vi "await_service_close.vi"(8 "error in (no error)":errorcluster, 11 "system.logging in":refnum<class "system.logging.lvclass">) -> (0 "error out":errorcluster, 3 "system.logging out":refnum<class "system.logging.lvclass">)   [LabVIEW 2021, in "system.logging.lvclass"]
uses:
  system.logging.lvclass
  system.logging.lvclass/system.logging.ctl
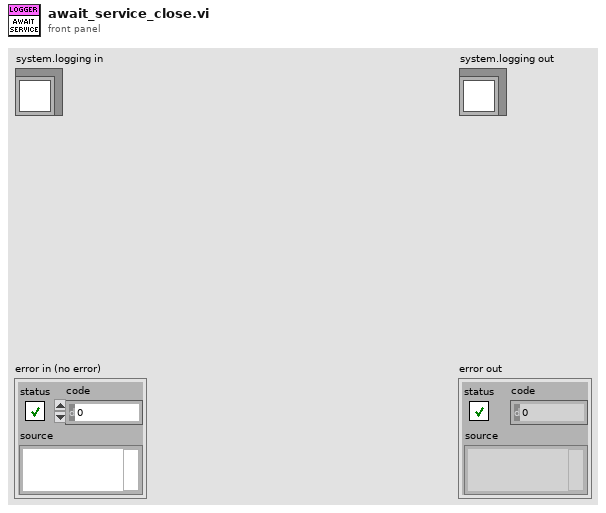
[diagram p1: front panel]
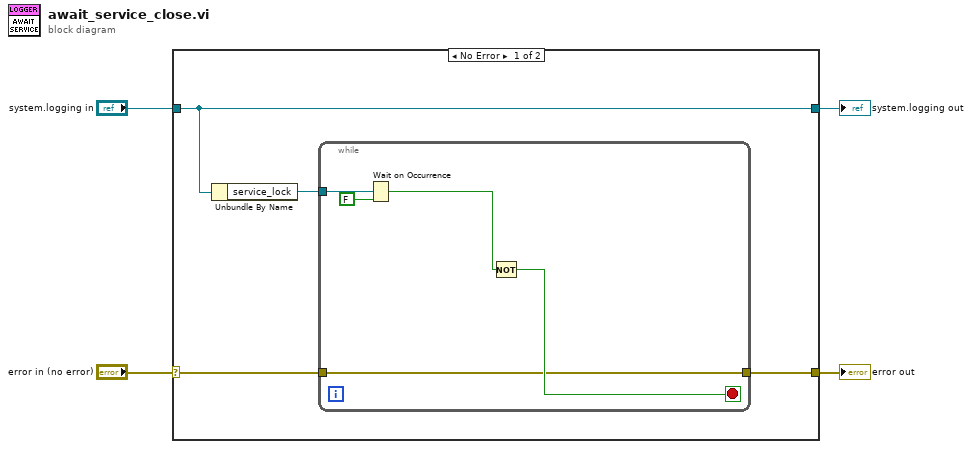
[diagram p0: block diagram]
diagram:
  n1 = case shown="No Error" "error in (no error)" {
    selector: "error in (no error)" -> [w6 w15]
    tunnel: [w5 w15] -> w3
    tunnel: [w8 w14] -> w1
    tunnel: "system.logging in" -> [w8 w14]
    frame No Error {
      n2 = Unbundle By Name(w8) -> ("service_lock"=w7:refnum<k4>)
      n3 = while {
        tunnel: w7 -> [w13]
        tunnel: w6 -> [w9]
        tunnel: [w9] -> w5
        stop <- w10 stop-if-true
        n4 = Wait on Occurrence(1:FALSE ("ignore previous (T)"), 2:w13) -> (0:w11:bool)  [unwired: 1 in]
        n5 = Not(x=w11) -> (.not. x?=w10:bool)
      }
    }
    frame Error {
    }
  }
  "error out" <- w3
  "system.logging out" <- w1
